vi "Initialise Front Panel.vi"(7 "This VI":refnum<vi>, 11 "UI Ref":T1) -> (0 "error out":errorcluster)   [LabVIEW 2021]
uses:
  Controls/UI Reference Cluster.ctl
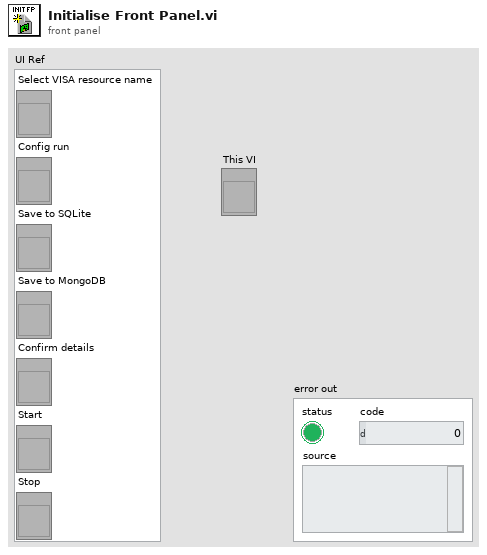
[diagram p1: front panel]
types:
  T1 = typedef "UI Reference Cluster.ctl" = cluster{"Select VISA resource name":refnum<vi>, "Config run":refnum<vi>, "Save to SQLite":refnum<vi>, "Save to MongoDB":refnum<vi>, "Confirm details":refnum<vi>, "Start":refnum<vi>, "Stop":refnum<vi>}
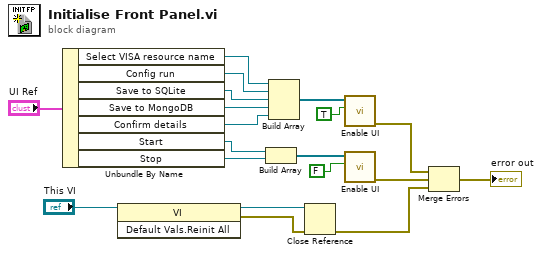
[diagram p0: block diagram]
diagram:
  n1 = Unbundle By Name("UI Ref") -> ("Select VISA resource name"=w14:refnum<vi>, "Config run"=w13:refnum<vi>, "Save to SQLite"=w12:refnum<vi>, "Save to MongoDB"=w11:refnum<vi>, "Confirm details"=w10:refnum<vi>, "Start"=w7:refnum<vi>, "Stop"=w6:refnum<vi>)
  n2 = invoke class="VI" method="Default Vals.Reinit All"(reference="This VI") -> (reference out=w17:refnum<vi>, error out=w16:errorcluster)  [unwired: 2 in, 1 out]
  n3 = Build Array(w7, w6) -> (w5:refnum<vi>[])
  n4 = Build Array(w14, w13, w12, w11, w10) -> (w9:refnum<vi>[])
  n5 = Close Reference(reference=w17, error in (no error)=w16) -> (error out=w15:errorcluster)
  n6 = call "Enable UI.vi"("Enable?"=TRUE, "output cluster"=w9) -> ("error out"=w2:errorcluster)  [unwired: 9 in]
  n7 = call "Enable UI.vi"("Enable?"=FALSE, "output cluster"=w5) -> ("error out"=w3:errorcluster)  [unwired: 9 in]
  n8 = Merge Errors(w2, w3, w15) -> (→"error out":errorcluster)
